vi "Reconnect.vi"(8 "error in (no error)":errorcluster, 11 "navX - SERIAL in":refnum<class "navX - SERIAL.lvclass">) -> (0 "error out":errorcluster, 3 "navX - SERIAL out":refnum<class "navX - SERIAL.lvclass">)   [LabVIEW 2015, in "navX Library v3.lvlib" / "navX - SERIAL.lvclass"]
uses:
  navX - SERIAL.lvclass
  navX - SERIAL.lvclass/navX - SERIAL.ctl
  navX - Interface/navX - Interface.lvclass
  _NI WPI Serial USB/_NI WPI Serial USB.lvlib
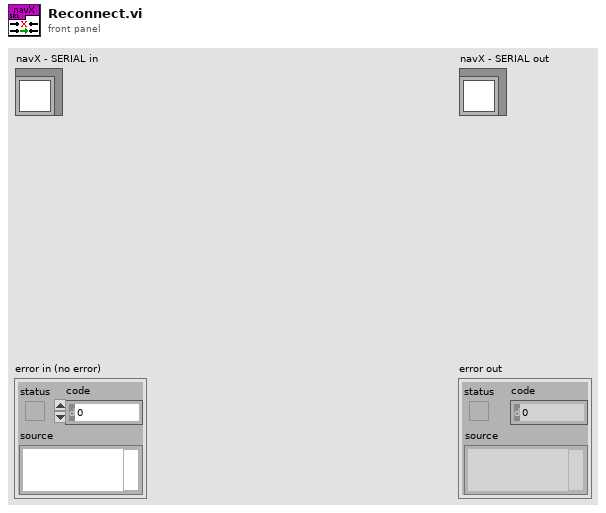
[diagram p1: front panel]
types:
  T1 = typedef "_NI WPI Serial USB.lvlib/WPI_SerialPort_USB.ctl" = enum16{"Onboard RS-232", "MXP TTL", "USB"}
  T2 = typedef "WPI_SerialPortRef.ctl" = cluster{"DevStatus":errorcluster, "Serial Port Name":refnum<visa-resource-name>}
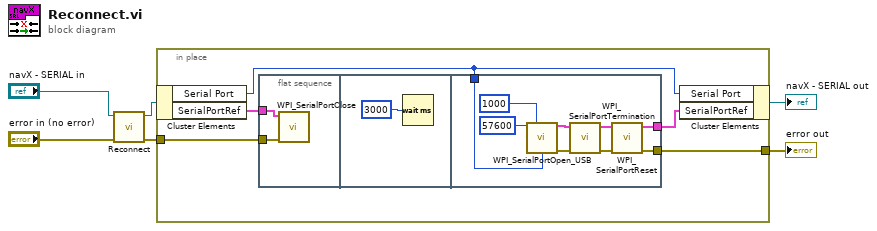
[diagram p0: block diagram]
diagram:
  n1 = call-parent "Reconnect.vi"("error in (no error)"="error in (no error)", "navX - Interface in"="navX - SERIAL in") -> ("error out"=w2:errorcluster, "navX - Interface out"=w4:refnum<class "navX - SERIAL.lvclass">)  [unwired: 8 in]
  n2 = in-place {
    in-place-border: [w10] -> w3
    in-place-border: w2 -> [w11]
    n3 = in-place-cluster #1(w4) -> ("Serial Port"=w9:T1, "SerialPortRef"=w8:T2)
    n4 = flat-sequence {
      tunnel: w11 -> [w12]
      tunnel: w8 -> [w13]
      tunnel: [w17] -> w10
      tunnel: [w16] -> w7
      tunnel: w9 -> [w15]
      frame #0 {
        n5 = call <vilib>:"WPI_SerialPortClose.vi"("error in (no error)"=w12, "SerialPortRef"=w13) -> ()  [unwired: 9 in, 1 out]
      }
      frame #1 {
        n6 = Wait (ms)(milliseconds to wait=u32 3000) -> ()  [unwired: 1 out]
      }
      frame #2 {
        n7 = call "WPI_SerialPortOpen_USB.vi"("Baud Rate"=u32 57600, "Timeout Value (ms)"=u32 1000, "Serial Port"=w15) -> ("SerialPortRef"=w18:T2, "error out"=w19:errorcluster)  [unwired: 11 in]
        n8 = call <vilib>:"WPI_SerialPortTermination.vi"("error in (no error)"=w19, "SerialPortRef"=w18) -> ("error out"=w20:errorcluster, "SerialPortRef"=w21:T2)  [unwired: 8 in]
        n9 = call <vilib>:"WPI_SerialPortReset.vi"("error in (no error)"=w20, "SerialPortRef"=w21) -> ("error out"=w17:errorcluster, "SerialPortRef"=w16:T2)  [unwired: 8 in]
      }
    }
    n10 = in-place-cluster #1("Serial Port"=w9, "SerialPortRef"=w7) -> (→"navX - SERIAL out":refnum<class "navX - SERIAL.lvclass">)
  }
  "error out" <- w3
